vi "WPI_DashboardLog NetworkTables2.vi"(6 "Robot IP":string, 8 "UDP Control":string, 9 "TCP":string, 10 "UDP Status":string) -> ()   [LabVIEW 2025]
uses:
  <vilib>/Rock Robotics/WPI/Dashboard/WPI_DashboardLoggingRecord.ctl
  <vilib>/Rock Robotics/WPI/Dashboard/WPI_DashboardNTL Header Type.ctl
  <vilib>/Rock Robotics/WPI/Dashboard/WPI_DashboardLogging Global.vi
  ntcoreffi.dll
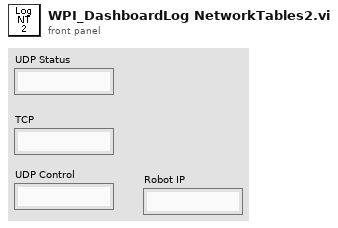
[diagram p1: front panel]
types:
  T1 = typedef "WPI_DashboardNTL Header Type.ctl" = cluster{"Version":i32, "Duration (ms)":i32, "TimeStamp":timestamp, "Robot IP":string, "Displays":string[]}
  T2 = typedef "WPI_DashboardLoggingRecord.ctl" = cluster{"time Ofst":i32, "video index":i32, "video index 2":i32, "video index 3":i32, "video index 4":i32, "UDP Status":string, "TCP":string, "UDP Control":string, "NT Updates":variant[]}
  T3 = enum16{"open", "replace", "create", "open or create", "replace or create", "replace or create with confirmation"}
  T4 = cluster{"Video 1":i32, "Video 2":i32, "Video 3":i32, "Video 4":i32}
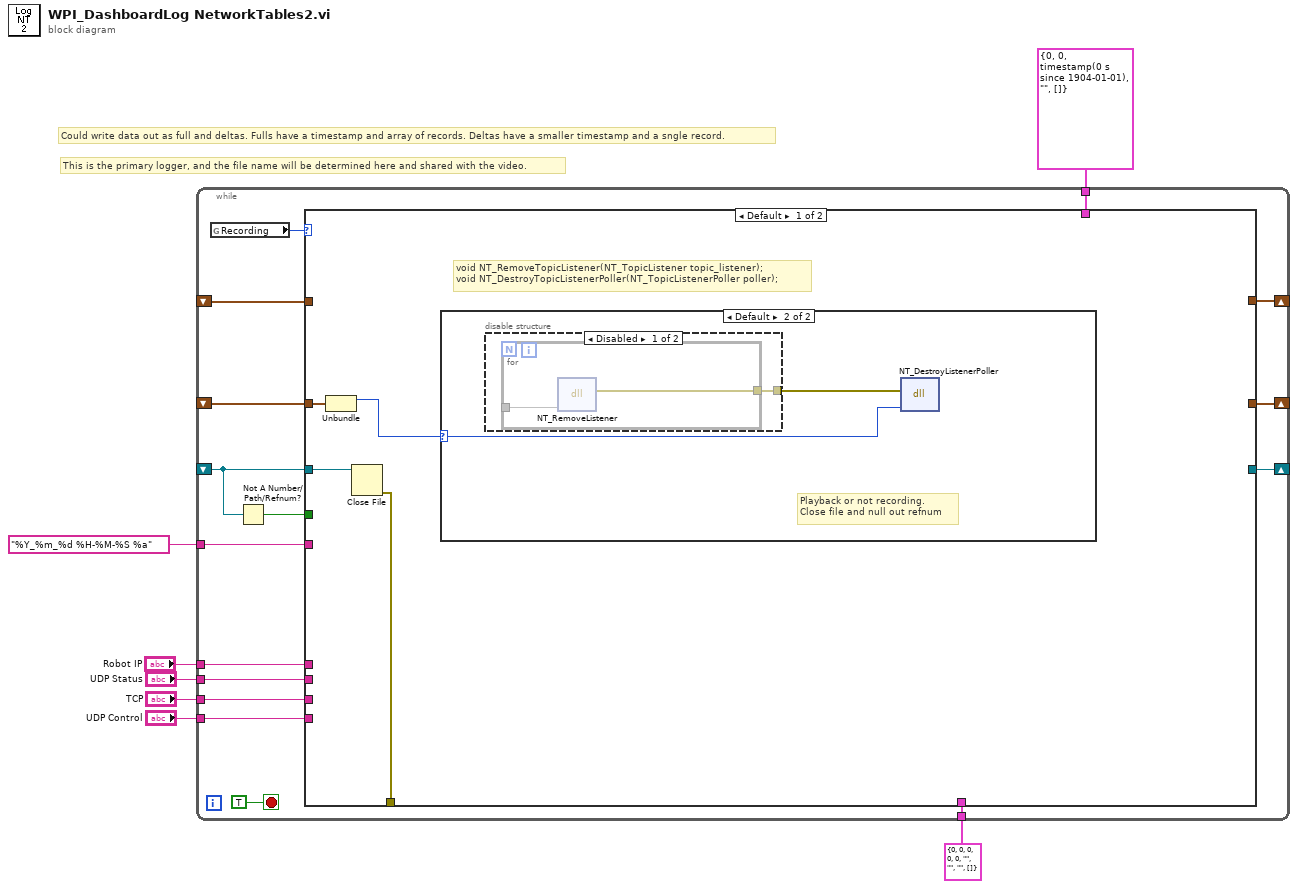
[diagram p0: block diagram]
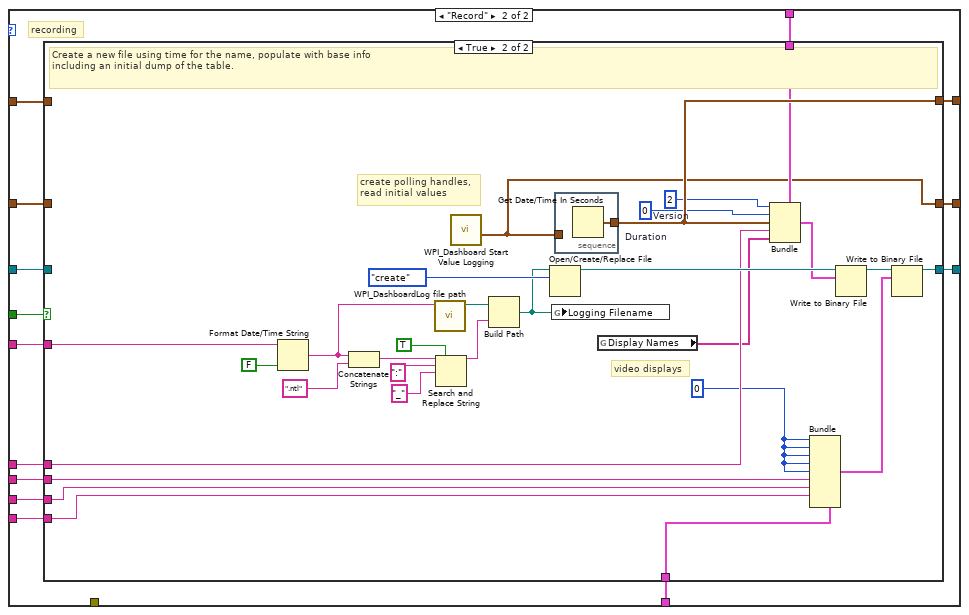
[diagram p4: hidden frame]
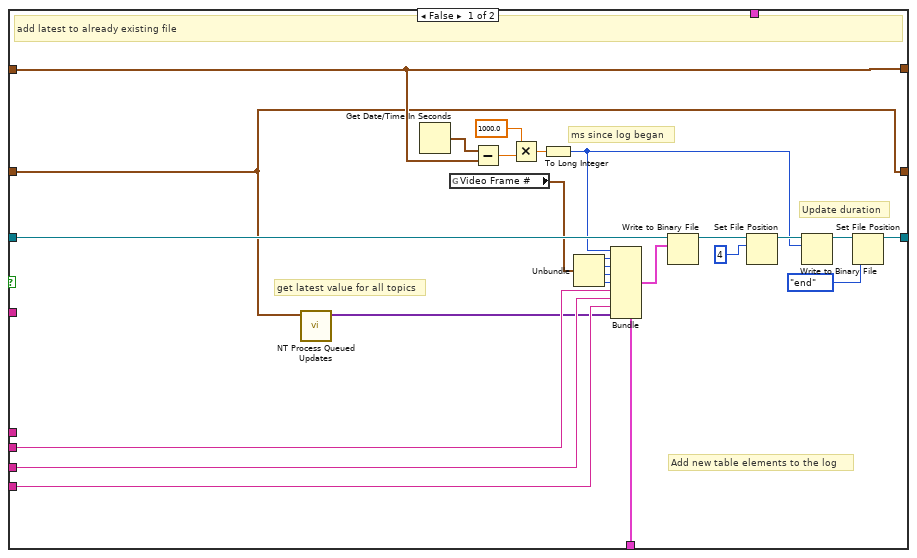
[diagram p5: hidden frame]
diagram:
  # "Could write data out as full and deltas. Fulls have a timestamp and array of records. Deltas have a smaller timestamp and a sngle record."
  # "This is the primary logger, and the file name will be determined here and shared with the video."
  n1 = while {
    shift-right: [w22] -> _
    shift-left: _ -> [w21]
    tunnel: "%Y_%m_%d %H-%M-%S %a" ("time format string (%c)") -> [w18]
    shift-right: [w17] -> _
    shift-left: _ -> [w16]
    tunnel: T2 {"time Ofst"=0, "video index"=0, "video index 2"=0, "video index 3"=0, "video index 4"=0, "UDP Status"="", "TCP"="", "UDP Control"="", "NT Updates"=[]} ("output cluster") -> [w15]
    tunnel: "UDP Status" -> [w14]
    tunnel: "TCP" -> [w13]
    tunnel: "UDP Control" -> [w12]
    tunnel: "Robot IP" -> [w11]
    tunnel: T1 {"Version"=0, "Duration (ms)"=0, "TimeStamp"=timestamp(0 s since 1904-01-01), "Robot IP"="", "Displays"=[]} ("Header") -> [w10]
    shift-right: [w8] -> _
    shift-left: _ -> [w9]
    stop <- TRUE stop-if-true
    n2 = global read "WPI_DashboardLogging Global.vi" "Recording"() -> (w19:enum32{"Stop", "Record", "Playback"})
    n3 = Not A Number/Path/Refnum?(number/path/refnum=w21) -> (NaN/Path/Refnum?=w20:bool)
    n4 = case shown="Default" w19 {
      tunnel: [_ w46] -> w22
      tunnel: w21 -> [w26 w45]
      tunnel: w20 -> [_ w44]
      tunnel: w18 -> [_ w43]
      tunnel: [_ w42] -> w17
      tunnel: w16 -> [_ w41]
      tunnel: [w27 _] -> _
      tunnel: w15 -> [_ w40]
      tunnel: w14 -> [_ w39]
      tunnel: w13 -> [_ w38]
      tunnel: w12 -> [_ w37]
      tunnel: w11 -> [_ w36]
      tunnel: w10 -> [_ w35]
      tunnel: w9 -> [w25 w33]
      tunnel: [_ w34] -> w8
      frame Default {
        # "void NT_RemoveTopicListener(NT_TopicListener topic_listener);\nvoid NT_DestroyTopicListenerPoller(NT_TopicListenerPoller poller);"
        n5 = Unbundle(w25) -> ("poller"=w24:u32)  [unwired: 1 out]
        n6 = Close File(refnum=w26) -> (error out=w27:errorcluster)  [unwired: 1 in, 1 out]
        n7 = case shown="Default" w24 {
          selector: w24 -> [_ w28]
          frame 0 {
          }
          frame Default {
            # "Playback or not recording.\nClose file and null out refnum"
            n8 = disable-structure shown="Disabled" {
              disable-tunnel: [w30 _] -> w29
              frame Disabled {
                n9 = for {
                  tunnel: [w32] -> w30
                  tunnel: _ -> [w31]
                  n10 = dll-call lib="ntcoreffi.*" fn="NT_RemoveListener"("listener"=w31) -> (error out=w32:errorcluster)  [unwired: 5 in, 1 out]
                }
              }
              frame Enabled {
              }
            }
            n11 = dll-call lib="ntcoreffi.*" fn="NT_DestroyListenerPoller"(error in=w29, "poller"=w28) -> ()  [unwired: 4 in, 2 out]
          }
        }
      }
      frame "Record" {
        # "recording"
        n12 = case shown="True" w44 {
          tunnel: [w69 w86] -> w46
          tunnel: w45 -> [w71 _]
          tunnel: w43 -> [_ w94]
          tunnel: [w70 w85] -> w42
          tunnel: w41 -> [w70 _]
          tunnel: w40 -> [w59 w82]
          tunnel: w39 -> [w57 w80]
          tunnel: w38 -> [w56 w79]
          tunnel: w37 -> [w55 w78]
          tunnel: w36 -> [_ w77]
          tunnel: w35 -> [_ w74]
          tunnel: [w47 w72] -> w34
          tunnel: w33 -> [w47 _]
          frame False {
            # "get latest value for all topics"
            # "Update duration"
            # "ms since log began"
            # "Add new table elements to the log"
            # "add latest to already existing file"
            n13 = call <vilib>:"NT Process Queued Updates.vi"("handles"=w47) -> ("Updates"=w48:variant[])  [unwired: 10 in]
            n14 = Get Date/Time In Seconds() -> (seconds since 1Jan1904=w68:timestamp)
            n15 = global read "WPI_DashboardLogging Global.vi" "Video Frame #"() -> (w53:T4)
            n16 = Subtract(x=w68, y=w70) -> (x-y=w67:dbl)
            n17 = Multiply(x=1000.0, y=w67) -> (x*y=w66:dbl)
            n18 = To Long Integer(number=w66) -> (32bit integer=w54:i32)
            n19 = Unbundle(w53) -> ("Video 1"=w52:i32, "Video 2"=w51:i32, "Video 3"=w50:i32, "Video 4"=w49:i32)
            n20 = Bundle(cluster=w59, "time Ofst"=w54, "video index"=w52, "video index 2"=w51, "video index 3"=w50, "video index 4"=w49, "UDP Status"=w57, "TCP"=w56, "UDP Control"=w55, "NT Updates"=w48) -> (w58:T2)
            n21 = Write to Binary File(file (use dialog)=w71, data=w58) -> (refnum out=w62:refnum<file>)  [unwired: 4 in, 2 out]
            n22 = Set File Position(offset (in bytes) (0)=i64 4, refnum=w62) -> (refnum out=w61:refnum<file>)  [unwired: 2 in, 1 out]
            n23 = Write to Binary File(file (use dialog)=w61, data=w54) -> (refnum out=w64:refnum<file>)  [unwired: 4 in, 2 out]
            n24 = Set File Position(refnum=w64, from (0:start)=enum16{"start", "end", "current"}."end") -> (refnum out=w69:refnum<file>)  [unwired: 2 in, 1 out]
          }
          frame True {
            w76 = 0
            w83 = 0  # Duration
            w84 = 2  # Version
            # "create polling handles,\nread initial values"
            # "video displays"
            # "Create a new file using time for the name, populate with base info\nincluding an initial dump of the table."
            n25 = Format Date/Time String(time format string (%c)=w94, UTC format=FALSE) -> (date/time string=w75:string)  [unwired: 1 in]
            n26 = Concatenate Strings(w75, ".ntl" ("time format string (%c)")) -> (w89:string)
            n27 = call <vilib>:"WPI_DashboardLog file path.vi"("Time Date String"=w75) -> ("appended path"=w100:path)  [unwired: 10 in]
            n28 = Search and Replace String(replace all?=TRUE ("replace all? (F)"), input string=w89, search string=":", replace string="_") -> (result string=w88:string)  [unwired: 4 in, 3 out]
            n29 = call <vilib>:"WPI_Dashboard Start Value Logging.vi"() -> ("handles"=w72:cluster{"poller":u32, "overAll Listener":u32})  [unwired: 10 in, 1 out]
            n30 = Build Path(base path=w100, name or relative path=w88) -> (appended path=w96:path)
            n31 = Open/Create/Replace File(file path (use dialog)=w96, operation (0:open)=T3."create") -> (refnum out=w98:refnum<file>)  [unwired: 4 in, 2 out]
            n32 = global write "WPI_DashboardLogging Global.vi" "Logging Filename"(w96) -> ()
            n33 = stacked-sequence {
              tunnel: [w101] -> w85
              tunnel: w72 -> [_]
              frame #0 {
                n34 = Get Date/Time In Seconds() -> (seconds since 1Jan1904=w101:timestamp)
              }
            }
            n35 = global read "WPI_DashboardLogging Global.vi" "Display Names"() -> (w73:string[])
            n36 = Bundle(cluster=w74, "Version"=w84, "Duration (ms)"=w83, "TimeStamp"=w85, "Robot IP"=w77, "Displays"=w73) -> (w97:T1)
            n37 = Bundle(cluster=w82, "time Ofst"=w76, "video index"=w76, "video index 2"=w76, "video index 3"=w76, "video index 4"=w76, "UDP Status"=w80, "TCP"=w79, "UDP Control"=w78) -> (w81:T2)  [unwired: 1 in]
            n38 = Write to Binary File(file (use dialog)=w98, data=w97) -> (refnum out=w87:refnum<file>)  [unwired: 4 in, 2 out]
            n39 = Write to Binary File(file (use dialog)=w87, data=w81) -> (refnum out=w86:refnum<file>)  [unwired: 4 in, 2 out]
          }
        }
      }
    }
  }
